vi "Channel.vi"(2 "number of samples":i32=300, 3 "error in":errorcluster, 4 "High & Low time":dbl=0.0001 format="%0.2e", 5 "counter":string="PXI1Slot5/ctr0") -> (0 "error out":errorcluster, 1 "task out":refnum<k21>)   [LabVIEW 2013]
uses:
  <vilib>/DAQmx/configure/timing.llb/DAQmx Timing (Implicit).vi
  <vilib>/DAQmx/create/channels.llb/DAQmx Create Channel (CO-Pulse Generation-Time).vi
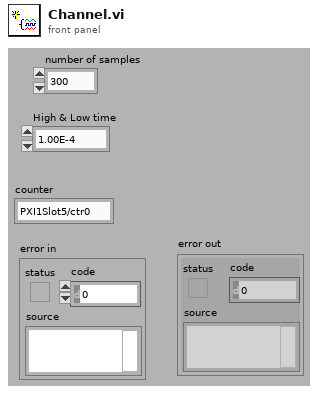
[diagram p1: front panel]
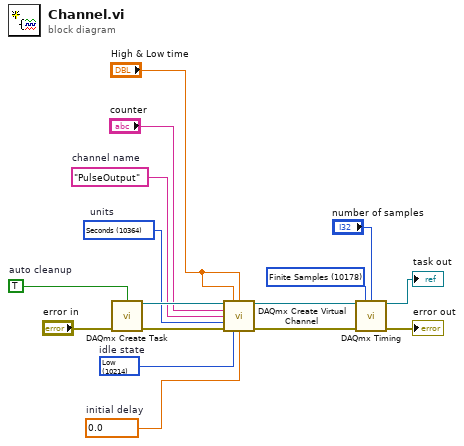
[diagram p0: block diagram]
diagram:
  w2 = 10178 items=["Finite Samples"=10178, "Continuous Samples"=10123, "Hardware Timed Single Point"=12522] ("sample mode")
  w7 = 0.0  # initial delay
  w8 = 10214 items=["High"=10192, "Low"=10214]  # idle state
  w9 = 10364 items=["Seconds"=10364, "From Custom Scale"=10065]  # units
  w10 = "PulseOutput"  # channel name
  w14 = TRUE  # auto cleanup
  n1 = call <vilib>:"DAQmx Create Task.vi"("auto cleanup"=w14, "error in"="error in") -> ("task out"=w13:refnum<k21>, "error out"=w15:errorcluster)  [unwired: 12 in]
  n2 = call-poly <vilib>:"DAQmx Create Virtual Channel.vi"("task in"=w13, "high time"="High & Low time", "low time"="High & Low time", "counter"="counter", "name to assign"=w10, "units"=w9, "error in"=w15, "idle state"=w8, "initial delay"=w7) -> ("task out"=w4:refnum<k21>, "error out"=w11:errorcluster)  [unwired: 5 in]
  n3 = call-poly <vilib>:"DAQmx Timing.vi"("task/channels in"=w4, "sample mode"=w2, "samples per channel"="number of samples", "error in"=w11) -> ("task out"=→"task out":refnum<k21>, "error out"=→"error out":errorcluster)  [unwired: 10 in]
